vi "Scoring logic.vi"(6 "Correct":cluster{"horizontal":i16, "vertical":i16}[](array[cluster]), 9 "x":T1, 10 "Coords":T1, 11 "Wrong":cluster{"horizontal":i16, "vertical":i16}[](array[cluster])) -> (1 "Checkbox":bool, 2 "Checkbox 2":bool, 3 "Checkbox 3":bool)   [LabVIEW 2021]
uses:
  <vilib>/Utility/miscctls.llb/LVPoint32TypeDef.ctl
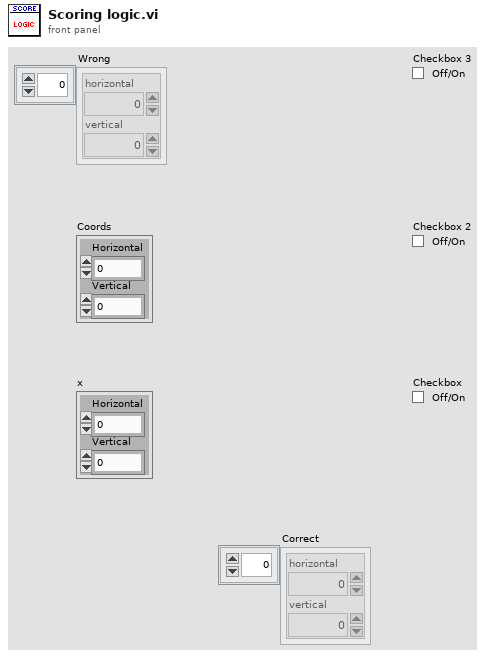
[diagram p1: front panel]
types:
  T1 = typedef "LVPoint32TypeDef.ctl" = cluster{"Horizontal":i32, "Vertical":i32}
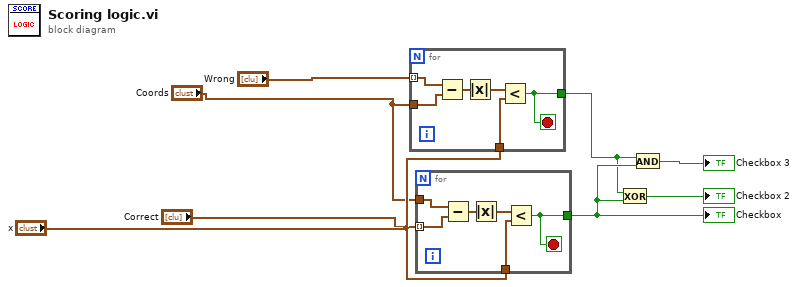
[diagram p0: block diagram]
diagram:
  n1 = for {
    tunnel: "Coords" -> [w13]
    tunnel: "Wrong" -> [w14] mode=indexing
    tunnel: "x" -> [w10]
    tunnel: [w9] -> w4
    stop <- w9 stop-if-true
    n2 = Subtract(x=w14, y=w13) -> (x-y=w12:T1)
    n3 = Absolute Value(x=w12) -> (abs(x)=w11:T1)
    n4 = Less?(x=w11, y=w10) -> (x < y?=w9:bool)
  }
  n5 = for {
    tunnel: "Correct" -> [w19] mode=indexing
    tunnel: "Coords" -> [w20]
    tunnel: "x" -> [w16]
    tunnel: [w15] -> w6
    stop <- w15 stop-if-true
    n6 = Subtract(x=w20, y=w19) -> (x-y=w18:T1)
    n7 = Absolute Value(x=w18) -> (abs(x)=w17:T1)
    n8 = Less?(x=w17, y=w16) -> (x < y?=w15:bool)
  }
  "Checkbox" <- w6
  n9 = Exclusive Or(1:w6, 2:w4) -> (0:→"Checkbox 2":bool)
  n10 = And(x=w4, y=w6) -> (x .and. y?=→"Checkbox 3":bool)
